vi "General Server.vi"(6 "Command Subscribe":bool, 7 "Connection":bool, 8 "error in (no error)":errorcluster, 10 "Server Status":string) -> (0 "last error":errorcluster, 2 "Received \nCommand":string)   [LabVIEW 2018]
uses:
  <vilib>/LabVIEW Open Source Project/MQTT Client/Client class/Client.lvclass/Client.ctl
  <vilib>/LabVIEW Open Source Project/MQTT Connection/MQTT_Base/Base Class/MQTT_Base.lvclass/MQTT_Base.ctl
  <vilib>/LabVIEW Open Source Project/Connection/Connection.TCP/Connection.TCP.lvclass
  C:/Program Files (x86)/National Instruments/LabVIEW 2018/vi.lib/LabVIEW Open Source Project/Connection/Connection/Connection.lvclass
  <vilib>/LabVIEW Open Source Project/MQTT Client/Client class/Client.lvclass
  C:/Program Files (x86)/National Instruments/LabVIEW 2018/vi.lib/LabVIEW Open Source Project/MQTT Connection/MQTT_Base/Base Class/MQTT_Base.lvclass
  <vilib>/LabVIEW Open Source Project/MQTT Control Packets/Control Packets/PUBLISH/PUBLISH.lvclass
  <vilib>/LabVIEW Open Source Project/MQTT Connection/MQTT_Base/Base Class/MQTT_Base.lvclass
  <vilib>/LabVIEW Open Source Project/Connection/Connection.LocalQueue/Connection.LocalQueue.lvclass
panel:
  in  "S4ICS_status":cluster{"id":i32, "message":string}
  in  "S4ICS_command":cluster{"id":i32, "message":string}
  in  "Stop Client":bool
  in  "Tab Control":enum32{"MQTT", "TCP/IP"}(tab)
  out "Command Payload":u8[](array[numeric]) format="%08b"
  in  "Command\nTopic Name":string="SPARC4 COMMAND"
  out "Unsuback":bool
  out "Suback":bool
  in  "clear command":bool
  out "Published":bool
  in  "Status\nTopic Name":string="SPARC4 STATUS"
  in  "broker address":string(combo)="test.mosquitto.org"
  # "S4ICS MESSENGER ENDPOINT"
  # "SERVER RECEIVED COMMAND"
  # "SERVER RESPONSE"
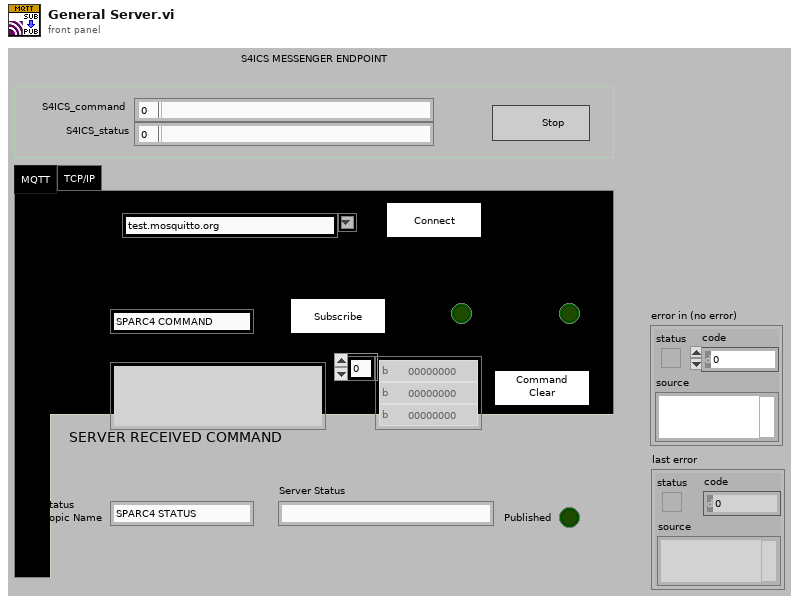
[diagram p1: front panel]
types:
  T1 = typedef "MQTT Client.lvlib/Client.lvclass/Public Events -- cluster.ctl" = cluster{"Connection Status":refnum<user-event>, "Connected":refnum<user-event>, "Application Message":refnum<user-event>}
  T2 = typedef "MQTT Base.lvlib/MQTT_Base.lvclass/Public Events -- cluster.ctl" = cluster{"Stop Event":refnum<user-event>, "Error Event":refnum<user-event>, "Inbound Message":refnum<user-event>}
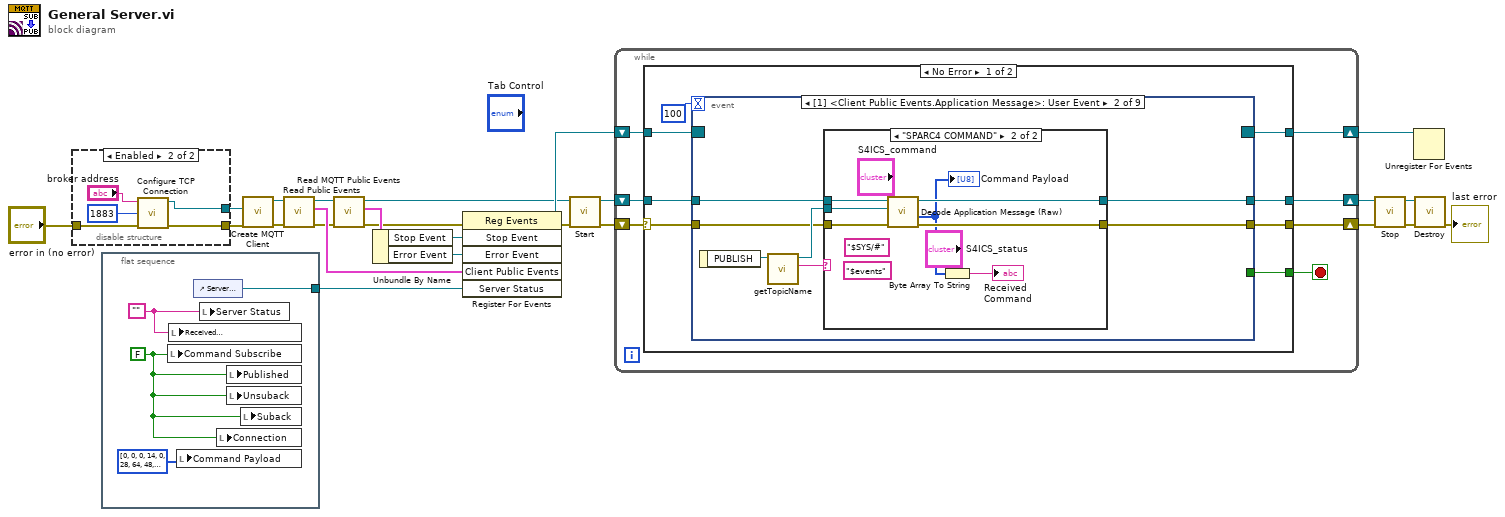
[diagram p0: block diagram]
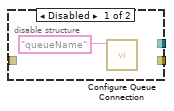
[diagram p2: hidden frame]
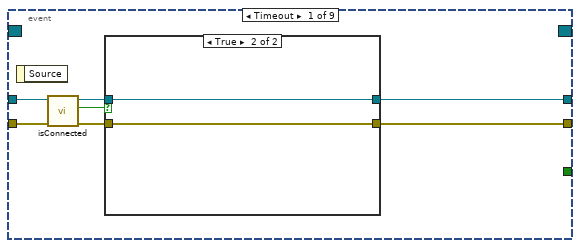
[diagram p3: hidden frame]
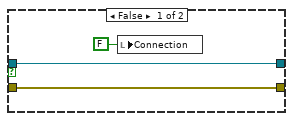
[diagram p4: hidden frame]
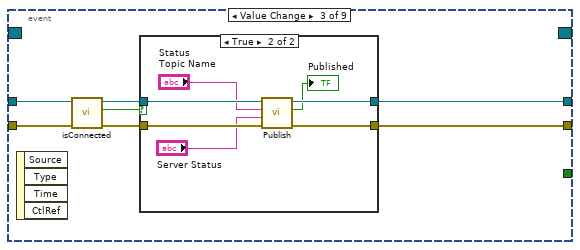
[diagram p6: hidden frame]
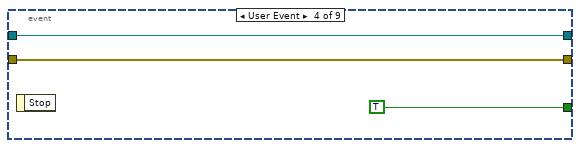
[diagram p8: hidden frame]
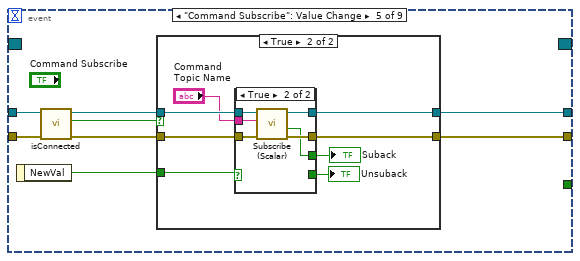
[diagram p9: hidden frame]
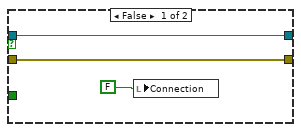
[diagram p10: hidden frame]
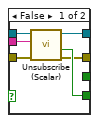
[diagram p11: hidden frame]
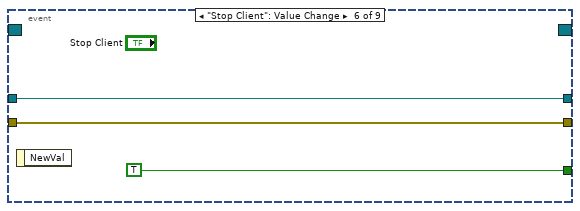
[diagram p12: hidden frame]
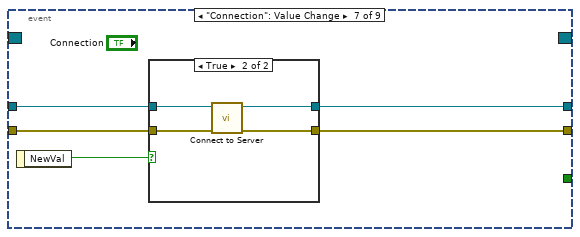
[diagram p13: hidden frame]
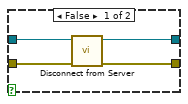
[diagram p14: hidden frame]
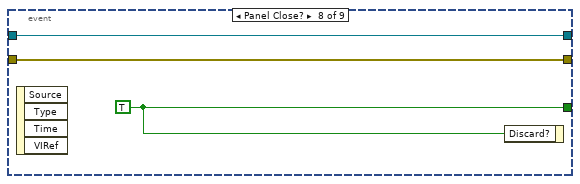
[diagram p15: hidden frame]
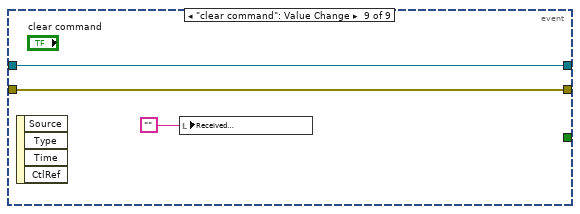
[diagram p16: hidden frame]
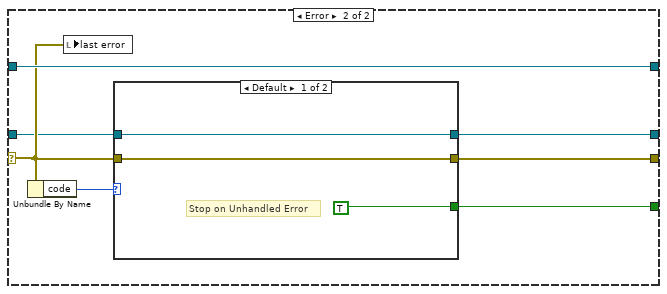
[diagram p17: hidden frame]
diagram:
  n1 = disable-structure shown="Enabled" {
    disable-tunnel: [_ w28] -> w3
    disable-tunnel: [_ w27] -> w2
    disable-tunnel: "error in (no error)" -> [_ w26]
    frame Disabled {
      n2 = call <vilib>:"Configure Queue Connection.vi"("Queue Name"="queueName") -> ()  [unwired: 9 in, 2 out]
    }
    frame Enabled {
      n3 = call <vilib>:"Configure TCP Connection.vi"("error in (no error)"=w26, "remote port (80)"=u16 1883, "address (localhost)"="broker address") -> ("error out"=w27:errorcluster, "Connection.TCP"=w28:refnum<class "Connection.TCP.lvclass">)  [unwired: 7 in]
    }
  }
  n4 = flat-sequence {
    tunnel: [w34] -> w4
    frame #0 {
      w31 = FALSE
      w33 = ""
      n5 = local write "Command Subscribe"(w31) -> ()
      n6 = local write "Received \nCommand"(w33) -> ()
      n7 = local write "Command Payload"(u8[] [0, 0, 0, 14, 0, 28, 64, 48, 255, 255, 255, 255, 18, 80, 117, 98, 108, 105, 115, 104, 105, 110, 103, 32, 67, 111, 109, 109, 97, 110, 100, 0, 0, 0, 0, 9, 73, 78, 73, 84, 32, 78, 79, 78, 69] ("Command Payload")) -> ()
      n8 = control-ref of="Server Status"() -> (w34:refnum<vi>)
      n9 = local write "Server Status"(w33) -> ()
      n10 = local write "Connection"(w31) -> ()
      n11 = local write "Published"(w31) -> ()
      n12 = local write "Unsuback"(w31) -> ()
      n13 = local write "Suback"(w31) -> ()
    }
  }
  n14 = call <vilib>:"Create MQTT Client.vi"("error in (no error)"=w2, "Connection Configuration"=w3) -> ("error out"=w7:errorcluster, "Client out"=w5:refnum<class "Client.lvclass">)  [unwired: 8 in]
  n15 = call <vilib>:"Read Public Events.vi"("error in (no error)"=w7, "Client in"=w5) -> ("error out"=w8:errorcluster, "Client Public Events"=w10:T1, "Client out"=w6:refnum<class "Client.lvclass">)  [unwired: 7 in]
  n16 = call <vilib>:"Read MQTT Public Events.vi"("error in (no error)"=w8, "MQTT_Base in"=w6) -> ("error out"=w9:errorcluster, "MQTT Public Events"=w17:T2, "MQTT_Base out"=w12:refnum<class "Client.lvclass">)  [unwired: 7 in]
  n17 = Unbundle By Name(w17) -> ("Stop Event"=w15:refnum<user-event>, "Error Event"=w16:refnum<user-event>)
  n18 = register-events(error in=w9, w15, w16, w10, w4) -> (reference out=w13:refnum<event-registration>, error out=w11:errorcluster)  [unwired: 1 in]
  n19 = call <vilib>:"Start.vi"("error in (no error)"=w11, "MQTT_Base in"=w12) -> ("error out"=w23:errorcluster, "MQTT_Base out"=w22:refnum<class "Client.lvclass">)  [unwired: 7 in, 1 out]
  n20 = while {
    shift-right: [w40] -> w14
    shift-left: w13 -> [w41]
    shift-right: [w37] -> w19
    shift-left: w22 -> [w38]
    shift-right: [w39] -> w21
    shift-left: w23 -> [w35]
    stop <- w36 stop-if-true
    n21 = case shown="No Error" w35 {
      selector: w35 -> [w42 w153]
      tunnel: w41 -> [w49 w156]
      tunnel: [w48 w156] -> w40
      tunnel: [w47 w151] -> w39
      tunnel: w38 -> [w45 w152]
      tunnel: [w44 w155] -> w37
      tunnel: [w43 w150] -> w36
      frame No Error {
        n22 = event shown="[1] <Client Public Events.Application Message>: User Event" {
          selector: w49 -> [_ _ _ _ _ _ _ _ _]
          dyn-events: [_ _ _ _ _ _ _ _ _] -> w48
          timeout: 100 -> [_ _ _ _ _ _ _ _ _]
          tunnel: w42 -> [w52 w65 w84 w96 w103 w129 w131 w144 w148]
          tunnel: [w55 w62 w79 w96 w99 w129 w132 w144 w148] -> w47
          tunnel: [_ _ _ TRUE _ TRUE _ w146 _] -> w43
          tunnel: w45 -> [w54 w66 w83 w94 w104 w130 w135 w145 w147]
          tunnel: [w56 w64 w78 w94 w98 w130 w133 w145 w147] -> w44
          event Timeout {
            n23 = event-data() -> ()  [unwired: 1 in, 1 out]
            n24 = call <vilib>:"isConnected.vi"("error in (no error)"=w52, "Client in"=w54) -> ("error out"=w51:errorcluster, "connected"=w50:bool, "Client out"=w53:refnum<class "Client.lvclass">)  [unwired: 7 in]
            n25 = case shown="True" w50 {
              tunnel: [w59 w61] -> w56
              tunnel: [w58 w60] -> w55
              tunnel: w53 -> [w59 w61]
              tunnel: w51 -> [w58 w60]
              frame False {
                n26 = local write "Connection"(FALSE ("Connection")) -> ()
              }
              frame True {
              }
            }
          }
          event User Event {
            n27 = event-data() -> ("PUBLISH"=w68:refnum<class "PUBLISH.lvclass">)  [unwired: 1 in]
            n28 = call <vilib>:"getTopicName.vi"("PUBLISH in"=w68) -> ("Topic"=w63:string, "PUBLISH out"=w67:refnum<class "PUBLISH.lvclass">)  [unwired: 8 in, 1 out]
            n29 = case shown="\"SPARC4 COMMAND\"" w63 {
              tunnel: w67 -> [_ w71]
              tunnel: w66 -> [w69 w77]
              tunnel: w65 -> [w70 w76]
              tunnel: [w69 w74] -> w64
              tunnel: [w70 w75] -> w62
              frame Default {
              }
              frame "SPARC4 COMMAND" {
                (unwired) "$events"
                (unwired) "$SYS/#" ("Topic Name")
                n30 = call <vilib>:"Decode Application Message (Raw).vi"("error in (no error)"=w76, "PUBLISH"=w71, "Client in"=w77) -> ("error out"=w75:errorcluster, "Payload"=w73:u8[], "Client out"=w74:refnum<class "Client.lvclass">)  [unwired: 5 in, 1 out]
                "Command Payload" <- w73
                n31 = Byte Array To String(unsigned byte array=w73) -> (string=→"Received \nCommand":string)
              }
            }
          }
          event Value Change {
            n32 = event-data() -> ()  [unwired: 1 in, 4 out]
            n33 = call <vilib>:"isConnected.vi"("error in (no error)"=w84, "Client in"=w83) -> ("error out"=w80:errorcluster, "connected"=w82:bool, "Client out"=w81:refnum<class "Client.lvclass">)  [unwired: 7 in]
            n34 = case shown="True" w82 {
              tunnel: w81 -> [w86 w93]
              tunnel: w80 -> [w85 w92]
              tunnel: [w85 w91] -> w79
              tunnel: [w86 w90] -> w78
              frame False {
              }
              frame True {
                n35 = call <vilib>:"Publish.vi"("error in (no error)"=w92, "Payload"="Server Status", "Topic Name (empty: Payload name)"="Status\nTopic Name", "Client in"=w93) -> ("error out"=w91:errorcluster, "Published"=→"Published":bool, "Client out"=w90:refnum<class "Client.lvclass">)  [unwired: 5 in]
              }
            }
          }
          event User Event {
            n36 = event-data() -> ()  [unwired: 1 in, 1 out]
          }
          event "Command Subscribe": Value Change {
            n37 = event-data() -> ("NewVal"=w97:bool)  [unwired: 1 in]
            n38 = call <vilib>:"isConnected.vi"("error in (no error)"=w103, "Client in"=w104) -> ("error out"=w100:errorcluster, "connected"=w102:bool, "Client out"=w101:refnum<class "Client.lvclass">)  [unwired: 7 in]
            n39 = case shown="True" w102 {
              tunnel: w101 -> [w105 w114]
              tunnel: w100 -> [w106 w115]
              tunnel: [w106 w110] -> w99
              tunnel: [w105 w109] -> w98
              tunnel: w97 -> [_ w108]
              frame False {
                n40 = local write "Connection"(FALSE ("Connection")) -> ()
              }
              frame True {
                n41 = case shown="True" w108 {
                  tunnel: [w116 w124] -> w109
                  tunnel: [w117 w123] -> w110
                  tunnel: w114 -> [w121 w127]
                  tunnel: w115 -> [w120 w126]
                  tunnel: "Command\nTopic Name" -> [w119 w125]
                  tunnel: [_ w122] -> w112
                  tunnel: [w118 _] -> w111
                  frame False {
                    n42 = call <vilib>:"Unsubscribe (Scalar).vi"("error in (no error)"=w120, "Topic Filter"=w119, "Client in"=w121) -> ("error out"=w117:errorcluster, "Ack"=w118:bool, "Client out"=w116:refnum<class "Client.lvclass">)  [unwired: 6 in]
                  }
                  frame True {
                    n43 = call <vilib>:"Subscribe (Scalar).vi"("error in (no error)"=w126, "Topic Filter"=w125, "Client in"=w127) -> ("error out"=w123:errorcluster, "Ack"=w122:bool, "Client out"=w124:refnum<class "Client.lvclass">)  [unwired: 6 in]
                  }
                }
                "Unsuback" <- w111
                "Suback" <- w112
              }
            }
          }
          event "Stop Client": Value Change {
            n44 = event-data() -> ()  [unwired: 1 in, 1 out]
          }
          event "Connection": Value Change {
            n45 = event-data() -> ("NewVal"=w134:bool)  [unwired: 1 in]
            n46 = case shown="True" w134 {
              tunnel: w135 -> [w139 w143]
              tunnel: [w138 w140] -> w133
              tunnel: [w137 w141] -> w132
              tunnel: w131 -> [w136 w142]
              frame False {
                n47 = call <vilib>:"Disconnect from Server.vi"("error in (no error)"=w136, "Client in"=w139) -> ("error out"=w137:errorcluster, "Client out"=w138:refnum<class "Client.lvclass">)  [unwired: 7 in, 1 out]
              }
              frame True {
                n48 = call <vilib>:"Connect to Server.vi"("error in (no error)"=w142, "Client in"=w143) -> ("error out"=w141:errorcluster, "Client out"=w140:refnum<class "Client.lvclass">)  [unwired: 6 in, 2 out]
              }
            }
          }
          event Panel Close? {
            w146 = TRUE
            n49 = event-data() -> ()  [unwired: 1 in, 4 out]
            n50 = event-data("Discard?"=w146) -> ()  [unwired: 1 in, 1 out]
          }
          event "clear command": Value Change {
            n51 = event-data() -> ()  [unwired: 1 in, 4 out]
            n52 = local write "Received \nCommand"("") -> ()
          }
        }
      }
      frame Error {
        n53 = Unbundle By Name(w153) -> ("code"=w154:i32)
        n54 = local write "last error"(w153) -> ()
        n55 = case shown="Default" w154 {
          tunnel: w152 -> [w159 w160]
          tunnel: [w159 w160] -> w155
          tunnel: w153 -> [w158 _]
          tunnel: [w158 _] -> w151
          tunnel: [TRUE _] -> w150
          frame Default {
            # "Stop on Unhandled Error"
          }
          frame 56, 63, 66 {
            # "Disconnected"
          }
        }
      }
    }
  }
  n56 = call <vilib>:"Stop.vi"("error in (no error)"=w21, "MQTT_Base in"=w19) -> ("error out"=w20:errorcluster, "MQTT_Base out"=w18:refnum<class "Client.lvclass">)  [unwired: 7 in, 1 out]
  n57 = Unregister For Events(event registration refnum=w14) -> ()  [unwired: 1 in, 1 out]
  n58 = call <vilib>:"Destroy.vi"("error in (no error)"=w20, "MQTT_Base in"=w18) -> ("error out"=→"last error":errorcluster)  [unwired: 8 in, 1 out]
